vi "systemLink Example.vi"   [LabVIEW 2019]
uses:
  Tag/Shared/typedefs/TagProperty.ctl
  Tag/Shared/typedefs/DataType.ctl
  Tag/Wrapper/Wrapper_class/Tag Value Cluster Wrapper.ctl
  Configuration/Configuration_class/NI Skyline Configuration.lvclass
  Tag/Shared/typedefs/Tag Value Cluster.ctl
  File/Filter/NI Skyline File Filter.lvclass
  File/HTTP/NI Skyline File HTTP.lvclass
  File/File/NI Skyline File.lvclass
  D:/Project/ARCOS-Code/builds/ARCOS-SDK/D/Project/ARCOS-Code/code-ARCOS-V4/UtilityVI/Skyline/File/Base/NI Skyline File Base.lvclass
  Tag/Wrapper/Wrapper AMQP_class/Open Tag AMQP.vi
  Tag/Wrapper/Wrapper_class/Read Tag History (DBL).vi
  Tag/Wrapper/Wrapper_class/Read Tag (DBL).vi
  Tag/Wrapper/Wrapper AMQP_class/Query Tags AMQP.vi
  Tag/Wrapper/Wrapper_class/Configure Retention (Duration).vi
  Tag/Wrapper/Wrapper_class/Close Tag (Multiple).vi
  Tag/Wrapper/Wrapper_class/Write Tag (DBL).vi
  Tag/Wrapper/Wrapper_class/Reset Aggregates (Single).vi
  Tag/Wrapper/Wrapper_class/Delete Tag (Single).vi
  Tag/Wrapper/Wrapper_class/Generate Tag Cluster (Timestamp) 2.vi
  Configuration/Configuration HTTP_class/Open Configuration HTTP Auto.vi
  File/File/Send File.vi
  File/File/Close (Single).vi
  File/File/Download (Sync) (Single).vi
  File/File/Delete (Single).vi
  File/File/Update Metadata Properties (Single).vi
  File/Filter/Create Filter (Extension).vi
  File/File/Query Files.vi
  Tag/Wrapper/History Window/Configure Tag History Window (Count).vi
  Message/AMQP/sync/Open (Sync).vi
  File/Auto Writable File/Send Packet (custom).vi
  File/Writable File/Send Last Packet (custom).vi
  File/File/Download (Async) (Single).vi
  Message/AMQP/NI Skyline Message AMQP (Sync).lvclass
  Configuration/Configuration HTTP_class/NI Skyline Configuration HTTP.lvclass
  Tag/Wrapper/Wrapper_class/NI Skyline Tag.lvclass
  Tag/Shared/NI Skyline Tag.lvlib
  Tag/Wrapper/Wrapper AMQP_class/NI Skyline Tag AMQP.lvclass
  Tag/Wrapper/History Window/NI Skyline Tag History Window.lvclass
  Message/NI Skyline Message.lvclass
  Utilities/NI Skyline Utilities.lvlib
  File/Base/NI Skyline File Base.lvclass
  File/Auto Writable File/NI Skyline Auto Writable File.lvclass
  File/Available File Event/NI Skyline Available File Event.lvclass
  File/Packet Event/NI Skyline File Packet Event.lvclass
  File/Writable File/NI Skyline Writable File.lvclass
  Configuration/Configuration AMQP_class/NI Skyline Configuration AMQP.lvclass
types:
  T1 = typedef "NI Skyline Tag.lvclass/Tag Value Cluster Wrapper.ctl" = cluster{"Configuration":refnum<class "NI Skyline Configuration.lvclass">, "Tag Cluster":T2}
  T2 = typedef "NI Skyline Tag.lvlib/Tag Value Cluster.ctl" = cluster{"Path":string, "Data Type":T3, "Value":string, "Time Stamp":timestamp}
  T3 = typedef "NI Skyline Tag.lvlib/DataType.ctl" = enum32{"Double", "I32", "String", "Boolean", "U64", "Timestamp"}
  T4 = typedef "NI Skyline Tag.lvlib/TagProperty.ctl" = cluster{"key":string, "value":string}
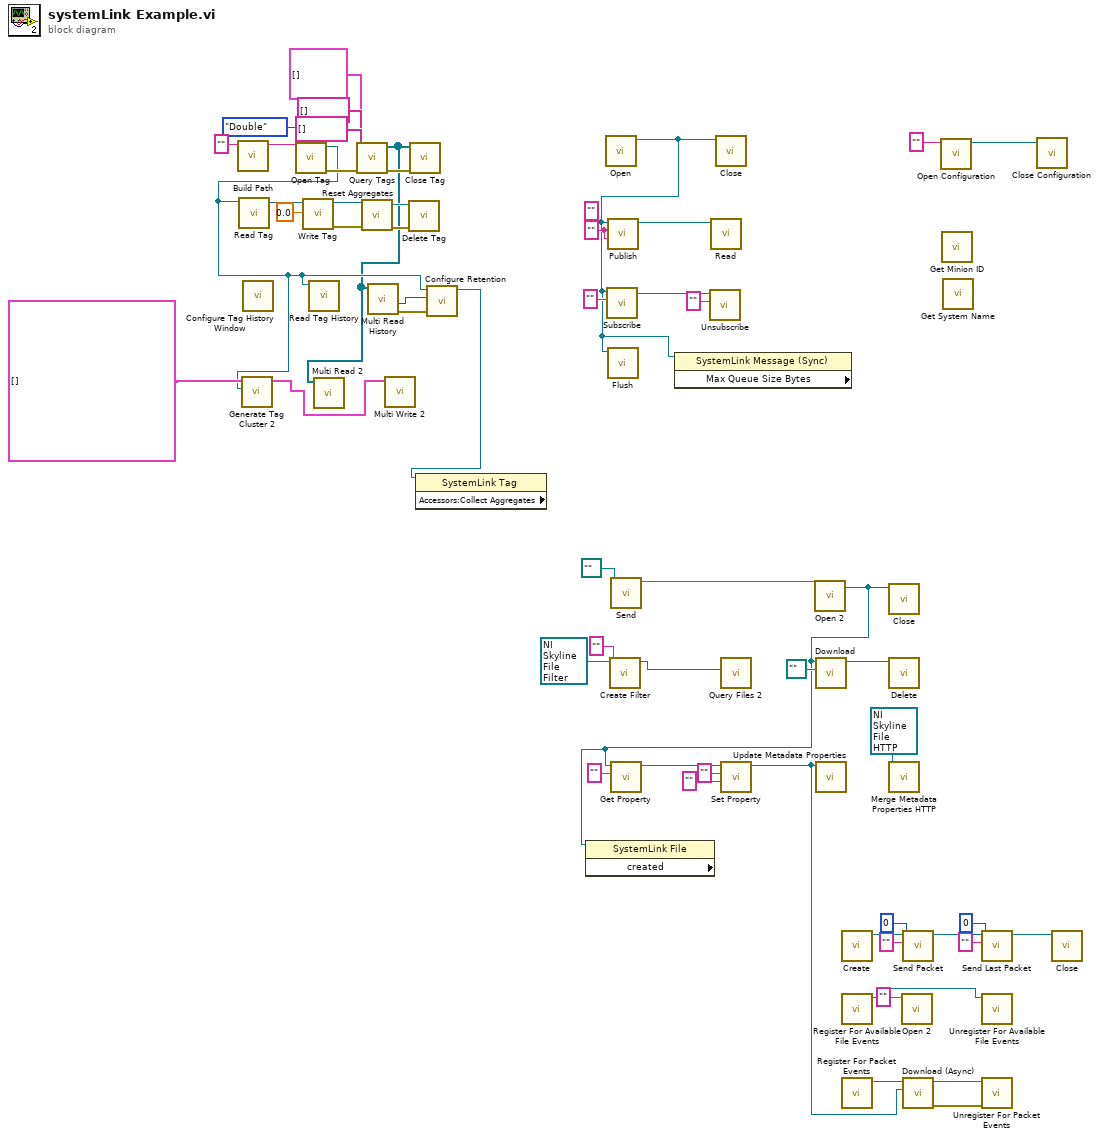
[diagram p0: block diagram]
diagram:
  (unwired) "" ("message")
  w31 = "" ("topic")
  n1 = call "Build Path.vi"("tag name"="") -> ("path"=w54:string)  [unwired: 10 in]
  n2 = call-poly "Configure Tag History Window.vi"() -> ()  [unwired: 11 in, 1 out]
  n3 = call-poly "Open Tag.vi"("data type"=DataType."Double", "path"=w54) -> ("error out"=w53:errorcluster, "tag"=w38:refnum<class "NI Skyline Tag.lvclass">)  [unwired: 8 in]
  n4 = call-poly "Read Tag.vi"("tag in"=w38) -> ("tag out"=w49:refnum<class "NI Skyline Tag.lvclass">)  [unwired: 6 in, 4 out]
  n5 = call-poly "Generate Tag Cluster 2.vi"("tag in"=w38, "tag clusters in"=T1[] []) -> ("tag clusters out"=w36:T1[])  [unwired: 7 in, 2 out]
  n6 = call-poly "Write Tag.vi"("value"=0.0, "tag in"=w49) -> ("error out"=w47:errorcluster, "tag out"=w46:refnum<class "NI Skyline Tag.lvclass">)  [unwired: 8 in]
  n7 = call-poly "Read Tag History.vi"("tag in"=w38) -> ()  [unwired: 6 in, 5 out]
  n8 = call-poly "Query Tags.vi"("error in (no error)"=w53, "properties"=T4[] [], "keywords"=string[] [], "paths"=string[] []) -> ("error out"=w42:errorcluster, "tags"=w37:refnum<class "NI Skyline Tag.lvclass">[])  [unwired: 5 in, 1 out]
  n9 = call "Multi Read 2.vi"("tags in"=w37) -> ()  [unwired: 8 in, 3 out]
  n10 = call-poly "Reset Aggregates.vi"("error in (no error)"=w47, "tag in"=w46) -> ("error out"=w44:errorcluster, "tag out"=w43:refnum<class "NI Skyline Tag.lvclass">)  [unwired: 8 in]
  n11 = call "Multi Read History.vi"("tags in"=w37) -> ("error out"=w41:errorcluster, "total count"=w40:i32)  [unwired: 7 in, 2 out]
  n12 = call "Multi Write 2.vi"("tag clusters"=w36) -> ()  [unwired: 10 in, 1 out]
  n13 = call-poly "Delete Tag.vi"("error in (no error)"=w44, "tag"=w43) -> ()  [unwired: 9 in, 1 out]
  n14 = call-poly "Close Tag.vi"("error in (no error)"=w42, "tags"=w37) -> ()  [unwired: 9 in, 1 out]
  n15 = call-poly "Configure Retention.vi"("error in (no error)"=w41, "days"=w40, "tag in"=w38) -> ("tag out"=w27:refnum<class "NI Skyline Tag.lvclass">)  [unwired: 7 in, 1 out]
  n16 = property on="Property Node" class="SystemLink Tag" props=["Accessors:Collect Aggregates"](reference=w27) -> ()  [unwired: 1 in, 3 out]
  n17 = call-poly "Open.vi"() -> ("message session"=w30:refnum<class "NI Skyline Message AMQP (Sync).lvclass">)  [unwired: 10 in, 1 out]
  n18 = call-dynamic "Subscribe.vi"("topic"="", "message session in"=w30) -> ("message session out"=w34:refnum<class "NI Skyline Message AMQP (Sync).lvclass">)  [unwired: 8 in, 1 out]
  n19 = call-dynamic "Publish.vi"("message"=w31, "topic"=w31, "message session in"=w30) -> ("message session out"=w35:refnum<class "NI Skyline Message AMQP (Sync).lvclass">)  [unwired: 7 in, 1 out]
  n20 = call-dynamic "Flush.vi"("sync message session in"=w30) -> ()  [unwired: 9 in, 2 out]
  n21 = call-poly "Create Filter.vi"("value"="", "filter in"=refnum<class "NI Skyline File Filter.lvclass"> refnum) -> ("filter out"=w22:refnum<class "NI Skyline File Filter.lvclass">)  [unwired: 8 in, 1 out]
  n22 = call-poly "Send.vi"("path"=path "") -> ("id"=w23:string)  [unwired: 8 in, 1 out]
  n23 = property class="SystemLink Message (Sync)" props=["Max Queue Size Bytes"](reference=w30) -> ()  [unwired: 1 in, 3 out]
  n24 = call-dynamic "Unsubscribe.vi"("topic"="", "message session in"=w34) -> ()  [unwired: 8 in, 2 out]
  n25 = call-dynamic "Read.vi"("sync message session in"=w35) -> ()  [unwired: 6 in, 5 out]
  n26 = call-dynamic "Close.vi"("message session"=w30) -> ()  [unwired: 10 in, 1 out]
  n27 = call-poly "Query Files 2.vi"("filter in"=w22) -> ()  [unwired: 8 in, 3 out]
  n28 = call-poly "Open 2.vi"("file id"=w23) -> ("file"=w4:refnum<class "NI Skyline File.lvclass">)  [unwired: 9 in, 1 out]
  n29 = property class="SystemLink File" props=["created"](reference=w4) -> ()  [unwired: 1 in, 3 out]
  n30 = call-dynamic "Get Property.vi"("key"="", "file in"=w4) -> ("file out"=w20:refnum<class "NI Skyline File.lvclass">)  [unwired: 6 in, 3 out]
  n31 = call-dynamic "Set Property.vi"("value"="", "key"="", "file in"=w20) -> ("file out"=w7:refnum<class "NI Skyline File.lvclass">)  [unwired: 7 in, 1 out]
  n32 = call-poly "Download.vi"("selected path"=path "", "file in"=w4) -> ("file out"=w21:refnum<class "NI Skyline File.lvclass">)  [unwired: 7 in, 2 out]
  n33 = call-poly "Update Metadata Properties.vi"("file in"=w7) -> ()  [unwired: 9 in, 2 out]
  n34 = call "Create.vi"() -> ("writable file"=w14:refnum<class "NI Skyline Auto Writable File.lvclass">)  [unwired: 9 in, 1 out]
  n35 = call "Register For Available File Events.vi"() -> ("available file event"=w8:refnum<class "NI Skyline Available File Event.lvclass">)  [unwired: 9 in, 2 out]
  n36 = call "Register For Packet Events.vi"() -> ("packet event"=w15:refnum<class "NI Skyline File Packet Event.lvclass">)  [unwired: 9 in, 2 out]
  n37 = call-poly "Close.vi"("file"=w4) -> ()  [unwired: 10 in, 1 out]
  n38 = call-poly "Delete.vi"("file"=w21) -> ()  [unwired: 10 in, 1 out]
  n39 = call "Merge Metadata Properties HTTP.vi"("file in"=refnum<class "NI Skyline File HTTP.lvclass"> refnum) -> ()  [unwired: 9 in, 2 out]
  n40 = call-poly "Open 2.vi"("file id"="") -> ()  [unwired: 9 in, 2 out]
  n41 = call-poly "Send Packet.vi"("packet number"=0, "data"="", "writable file in"=w14) -> ("writable file out"=w11:refnum<class "NI Skyline Writable File.lvclass">)  [unwired: 6 in, 2 out]
  n42 = call-poly "Download (Async).vi"("file in"=w7, "packet event in"=w15) -> ("error out"=w26:errorcluster, "packet event out"=w25:refnum<class "NI Skyline File Packet Event.lvclass">)  [unwired: 6 in, 2 out]
  n43 = call-poly "Open Configuration.vi"("configuration id"="" ("configuration id (default)")) -> ("configuration"=w28:refnum<class "NI Skyline Configuration HTTP.lvclass">)  [unwired: 9 in, 1 out]
  n44 = call "Get Minion ID.vi"() -> ()  [unwired: 11 in, 1 out]
  n45 = call "Get System Name.vi"() -> ()  [unwired: 11 in, 1 out]
  n46 = call-poly "Send Last Packet.vi"("packet number"=0, "data"="", "writable file in"=w11) -> ("file out"=w10:refnum<class "NI Skyline File.lvclass">)  [unwired: 7 in, 1 out]
  n47 = call "Unregister For Available File Events.vi"("available file event"=w8) -> ()  [unwired: 10 in, 1 out]
  n48 = call "Unregister For Packet Events.vi"("error in (no error)"=w26, "packet event"=w25) -> ()  [unwired: 9 in, 1 out]
  n49 = call-dynamic "Close Configuration.vi"("configuration"=w28) -> ()  [unwired: 10 in, 1 out]
  n50 = call-poly "Close.vi"("file"=w10) -> ()  [unwired: 10 in, 1 out]
